vi "getI.vi"(1 "P":dbl format="%#_13g", 2 "param":T1={"Srated"=25000.0, "eta [pu]"=0.99, "Eeq"=3.0, "Zeq"=260.0} {"Zeq" format="%#_13g"; "Eeq" format="%#_13g"; "eta [pu]" format="%#_13g"}) -> (0 "I":dbl)   [LabVIEW 2021]
panel:
  out "V":dbl
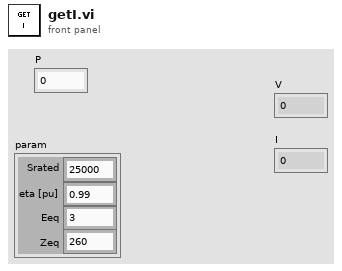
[diagram p1: front panel]
types:
  T1 = cluster{"Srated":dbl, "eta [pu]":dbl, "Eeq":dbl, "Zeq":dbl}
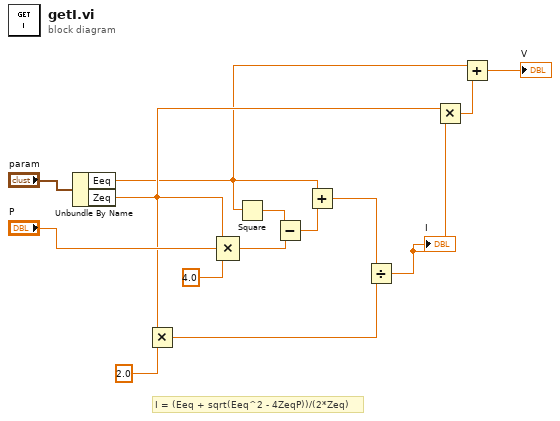
[diagram p0: block diagram]
diagram:
  # "I = (Eeq + sqrt(Eeq^2 - 4ZeqP))/(2*Zeq)"
  n1 = Unbundle By Name("param") -> ("Eeq"=w2:dbl, "Zeq"=w4:dbl)
  n2 = Multiply(x=w4, y=2.0 ("value")) -> (x*y=w6:dbl)
  n3 = Compound Arithmetic op=MULTIPLY(w4, "P", 4.0 ("value")) -> (w11:dbl)
  n4 = Square(x=w2) -> (x^2=w10:dbl)
  n5 = Subtract(x=w10, y=w11) -> (x-y=w9:dbl)
  n6 = Add(x=w2, y=w9) -> (x+y=w8:dbl)
  n7 = Divide(x=w8, y=w6) -> (x/y=w5:dbl)
  "I" <- w5
  n8 = Multiply(x=w4, y=w5) -> (x*y=w3:dbl)
  n9 = Add(x=w2, y=w3) -> (x+y=→"V":dbl)
